vi "GetChildByIndex.vi"(8 "error in (no error)":errorcluster, 10 "Index(0)":i32, 11 "BrowerComposite in":refnum<class "BrowerComposite.lvclass">) -> (0 "error out":errorcluster, 2 "BrowerComponent":refnum<class "BrowerComponent.lvclass">, 3 "BrowerComposite out":refnum<class "BrowerComposite.lvclass">)   [LabVIEW 2015, in "BrowerComposite.lvclass"]
uses:
  BrowerComposite.lvclass
  BrowerComponent/BrowerComponent.lvclass
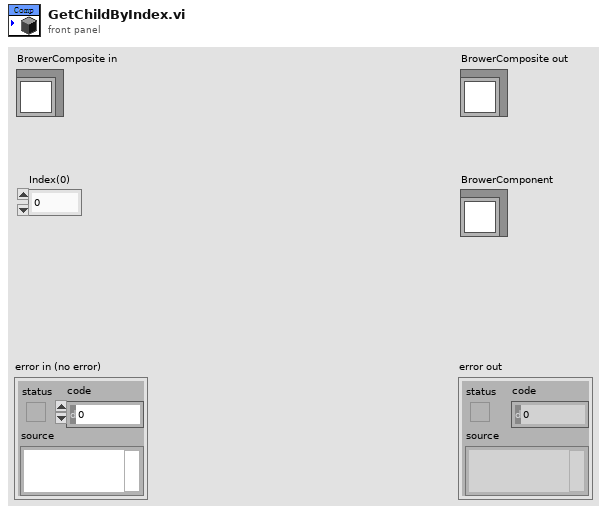
[diagram p1: front panel]
types:
  T1 = typedef "BrowerComposite.lvclass/ObjectAttributes.ctl" = cluster{"BrowerComponents":refnum<class "BrowerComponent.lvclass">[], "BrowerComponentIDs":string[]}
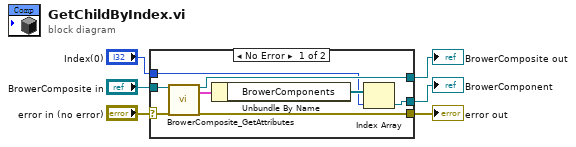
[diagram p0: block diagram]
diagram:
  n1 = case shown="No Error" "error in (no error)" {
    selector: "error in (no error)" -> [w8 w15]
    tunnel: "BrowerComposite in" -> [w14 w16]
    tunnel: "Index(0)" -> [w10 _]
    tunnel: [w11 w16] -> w3
    tunnel: [w9 _] -> w2
    tunnel: [w7 w15] -> w1
    frame No Error {
      n2 = call "BrowerComposite_GetAttributes.vi"("reference in"=w14, "error in (no error)"=w8) -> ("reference out"=w11:refnum<class "BrowerComposite.lvclass">, "Data"=w13:T1, "error out"=w7:errorcluster)  [unwired: 14 in, 1 out]
      n3 = Unbundle By Name(w13) -> ("BrowerComponents"=w12:refnum<class "BrowerComponent.lvclass">[])
      n4 = Index Array(array=w12, index=w10) -> (element=w9:refnum<class "BrowerComponent.lvclass">)
    }
    frame Error {
    }
  }
  "error out" <- w1
  "BrowerComposite out" <- w3
  "BrowerComponent" <- w2
